vi "Three-PID.vi"(7 "Reset":bool, 8 "Error In":errorcluster, 11 "目標角度":dbl[](array[numeric])) -> (0 "Error Out":errorcluster)   [LabVIEW 2019]
uses:
  <vilib>/addons/control/pid/pid.llb/PID (DBL Array).vi
  <vilib>/addons/control/pid/NI_PID_pid.lvlib
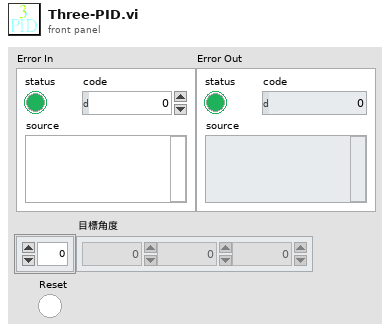
[diagram p1: front panel]
types:
  T1 = cluster{"proportional gain (Kc)":dbl, "integral time (Ti, min)":dbl, "derivative time (Td, min)":dbl}[]
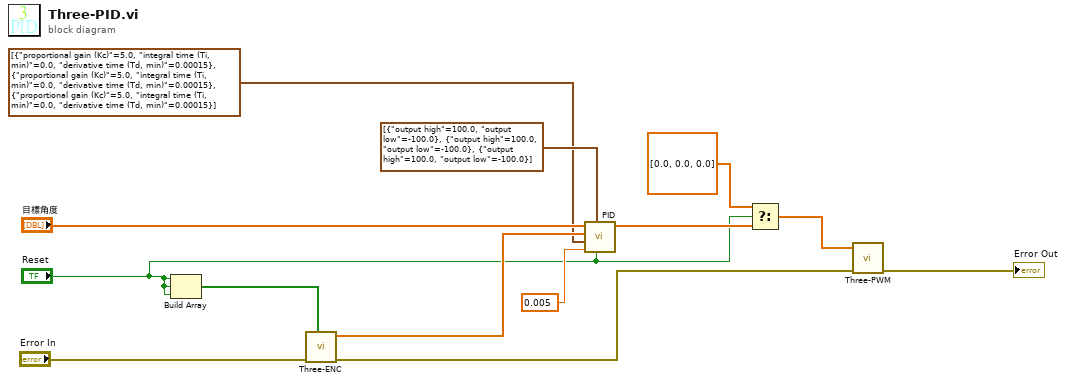
[diagram p0: block diagram]
diagram:
  n1 = Build Array("Reset", "Reset", "Reset") -> (w5:bool[])
  n2 = call "Three-ENC.vi"("Reset"=w5, "Error In"="Error In") -> ("Error Out"=w2:errorcluster, "Counter Value"=w12:dbl[])  [unwired: 8 in]
  n3 = call-poly <vilib>:"PID.vi"("reinitialize? (F)"="Reset", "output range"=cluster{"output high":dbl, "output low":dbl}[] [{"output high"=100.0, "output low"=-100.0}, {"output high"=100.0, "output low"=-100.0}, {"output high"=100.0, "output low"=-100.0}], "dt (s)"=0.005, "PID gains"=T1 [{"proportional gain (Kc)"=5.0, "integral time (Ti, min)"=0.0, "derivative time (Td, min)"=0.00015}, {"proportional gain (Kc)"=5.0, "integral time (Ti, min)"=0.0, "derivative time (Td, min)"=0.00015}, {"proportional gain (Kc)"=5.0, "integral time (Ti, min)"=0.0, "derivative time (Td, min)"=0.00015}], "process variable"=w12, "setpoint"="目標角度") -> ("output"=w7:dbl[])  [unwired: 4 in, 1 out]
  n4 = Select(t=dbl[] [0.0, 0.0, 0.0], s="Reset", f=w7) -> (s? t:f=w3:dbl[])
  n5 = call "Three-PWM.vi"("Error In"=w2, "Dutycycle(%)"=w3) -> ("Error Out"=→"Error Out":errorcluster)  [unwired: 9 in]
